vi "postData_bkp.vi"(7 "LabVIEW Web Service Request":refnum<class "Web Request.lvclass">) -> (2 "Result":string)   [LabVIEW 2016]
uses:
  <vilib>/wsapi/Web Request.lvclass
  <vilib>/Utility/file.llb/Read Delimited Spreadsheet (string).vi
  <vilib>/Utility/file.llb/Write Delimited Spreadsheet (string).vi
  <vilib>/Utility/file.llb/Read Delimited Spreadsheet (DBL).vi
  <vilib>/Utility/file.llb/Write Delimited Spreadsheet (DBL).vi
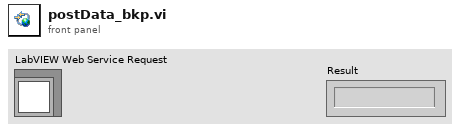
[diagram p1: front panel]
types:
  T1 = enum16{"open", "replace", "create", "open or create", "replace or create", "replace or create with confirmation"}
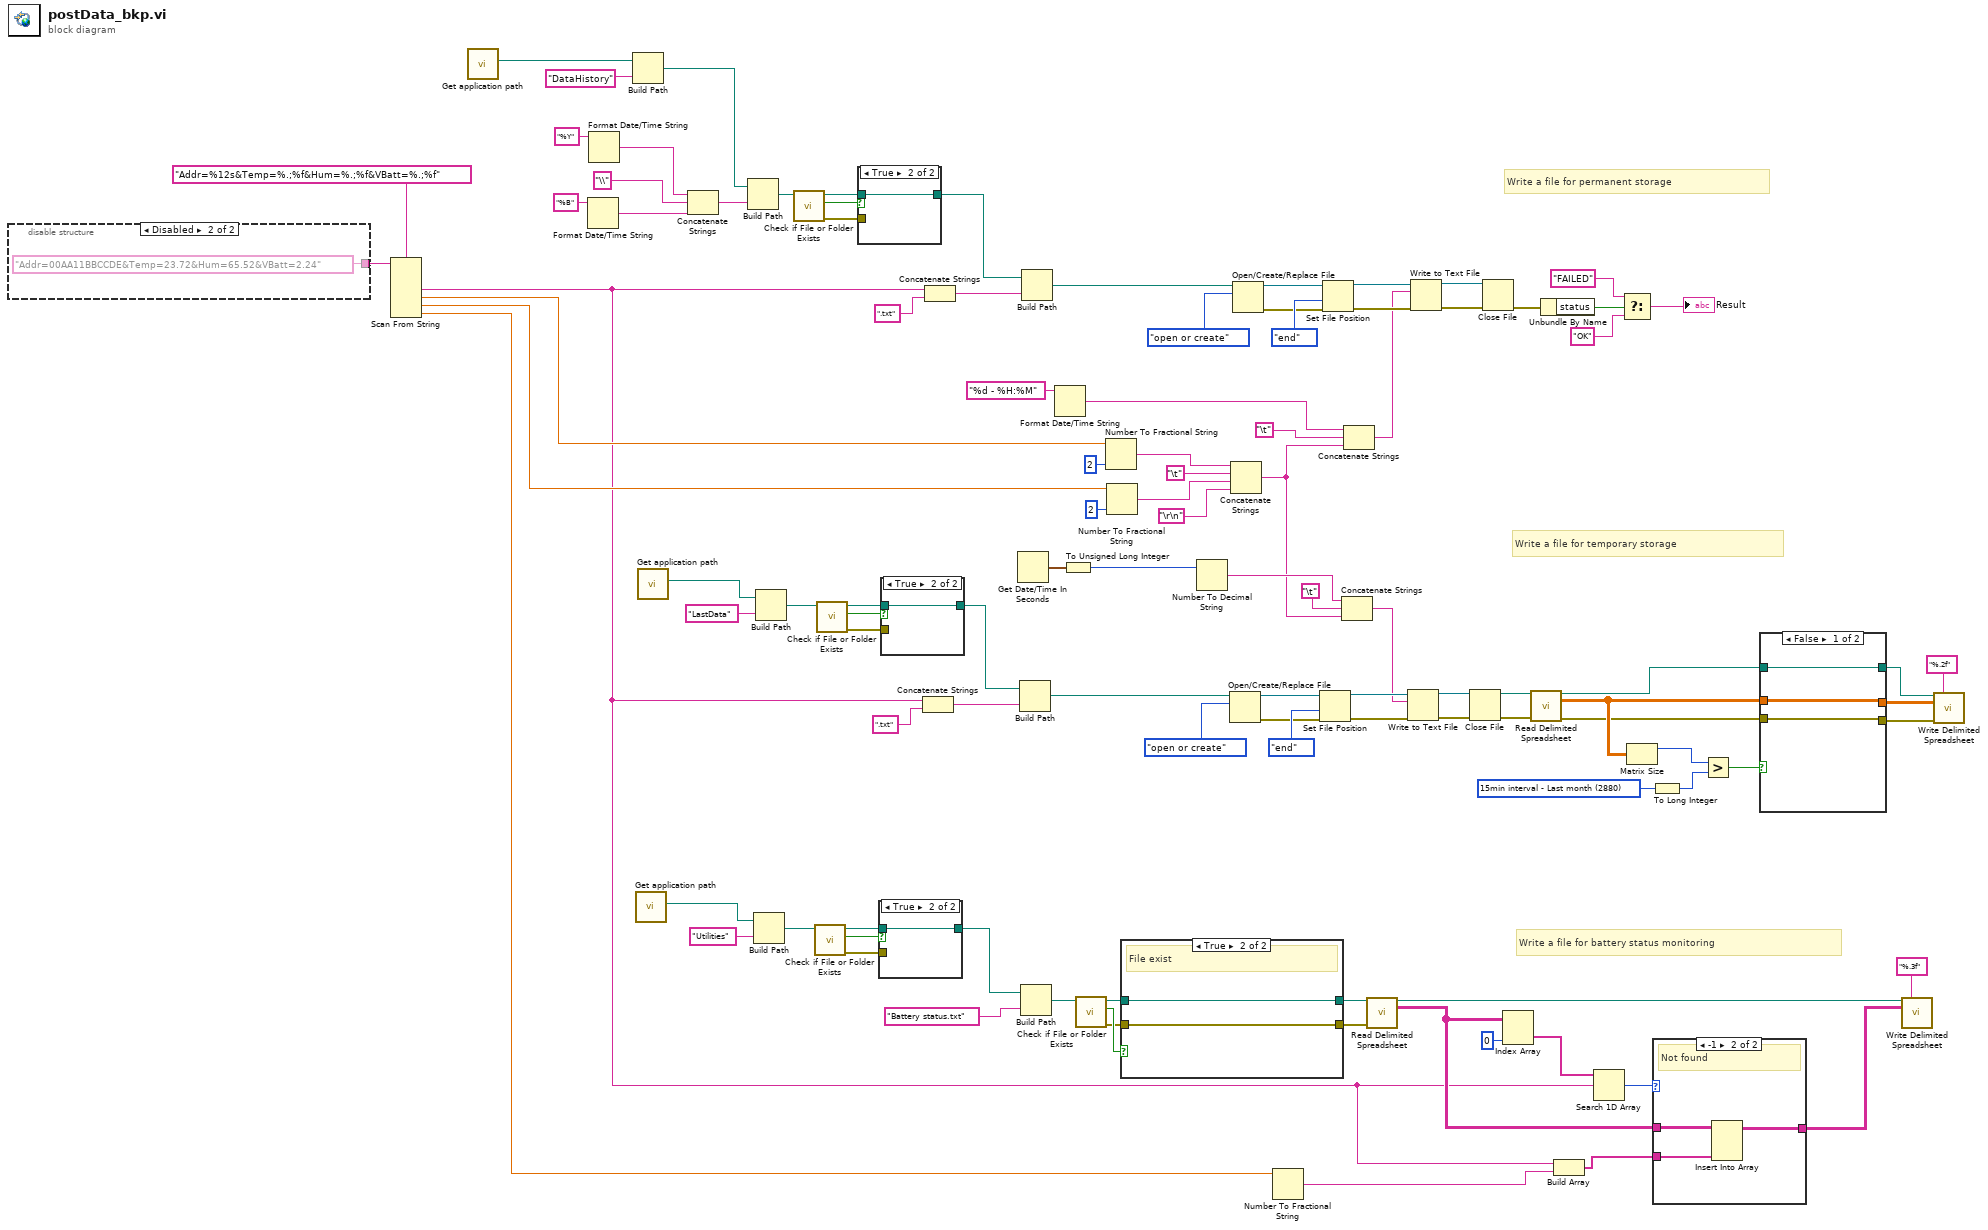
[diagram p0: block diagram]
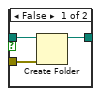
[diagram p2: hidden frame]
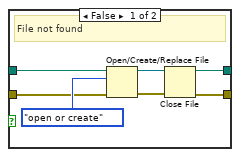
[diagram p3: hidden frame]
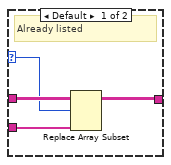
[diagram p4: hidden frame]
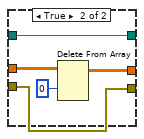
[diagram p5: hidden frame]
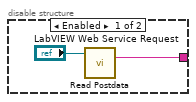
[diagram p6: hidden frame]
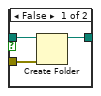
[diagram p7: hidden frame]
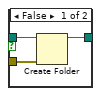
[diagram p8: hidden frame]
diagram:
  w11 = u16 2880 items=["5min interval - Last week"=2016, "5min interval - Last month"=8640, "10min interval - Last week"=1008, "10min interval - Last month"=4320, "15min interval - Last week"=672, "15min interval - Last month"=2880]
  # "Write a file for battery status monitoring"
  # "Write a file for temporary storage"
  # "Write a file for permanent storage"
  n1 = disable-structure shown="Disabled" {
    disable-tunnel: [w107 "Addr=00AA11BBCCDE&Temp=23.72&Hum=65.52&VBatt=2.24" ("input string")] -> w35
    frame Enabled {
      n2 = call <vilib>:"Read Postdata.vi"("LabVIEW Web Service Request"="LabVIEW Web Service Request") -> ("postdata"=w107:string)  [unwired: 12 in, 2 out]
    }
    frame Disabled {
    }
  }
  n3 = Scan From String(format string="Addr=%12s&Temp=%.;%f&Hum=%.;%f&VBatt=%.;%f", input string=w35) -> (output 1=w23:string, output 2=w88:dbl, output 3=w87:dbl, output 4=w22:dbl)  [unwired: 6 in, 3 out]
  n4 = call "Get application path.vi"() -> ("Application path"=w31:path)  [unwired: 11 in]
  n5 = Format Date/Time String(time format string (%c)="%B") -> (date/time string=w82:string)  [unwired: 2 in]
  n6 = Format Date/Time String(time format string (%c)="%Y") -> (date/time string=w84:string)  [unwired: 2 in]
  n7 = Build Path(base path=w31, name or relative path="DataHistory") -> (appended path=w34:path)
  n8 = call "Get application path.vi"() -> ("Application path"=w2:path)  [unwired: 11 in]
  n9 = call "Get application path.vi"() -> ("Application path"=w30:path)  [unwired: 11 in]
  n10 = Concatenate Strings(w84, "\\" ("string"), w82) -> (w89:string)
  n11 = Build Path(base path=w34, name or relative path=w89) -> (appended path=w80:path)
  n12 = Build Path(base path=w2, name or relative path="Utilities") -> (appended path=w7:path)
  n13 = Build Path(base path=w30, name or relative path="LastData") -> (appended path=w72:path)
  n14 = call <vilib>:"Check if File or Folder Exists.vi"("path"=w80) -> ("error out"=w79:errorcluster, "file or folder exists?"=w77:bool, "dup path"=w78:path)  [unwired: 8 in]
  n15 = call <vilib>:"Check if File or Folder Exists.vi"("path"=w7) -> ("error out"=w6:errorcluster, "file or folder exists?"=w4:bool, "dup path"=w5:path)  [unwired: 8 in]
  n16 = call <vilib>:"Check if File or Folder Exists.vi"("path"=w72) -> ("error out"=w71:errorcluster, "file or folder exists?"=w69:bool, "dup path"=w70:path)  [unwired: 8 in]
  n17 = case shown="True" w77 {
    tunnel: w79 -> [w112 _]
    tunnel: w78 -> [w111 w113]
    tunnel: [w110 w113] -> w76
    frame False {
      n18 = Create Folder(path (use dialog)=w111, error in=w112) -> (created path=w110:path)  [unwired: 1 in, 2 out]
    }
    frame True {
    }
  }
  n19 = case shown="True" w4 {
    tunnel: w6 -> [w116 _]
    tunnel: w5 -> [w115 w117]
    tunnel: [w114 w117] -> w1
    frame False {
      n20 = Create Folder(path (use dialog)=w115, error in=w116) -> (created path=w114:path)  [unwired: 1 in, 2 out]
    }
    frame True {
    }
  }
  n21 = case shown="True" w69 {
    tunnel: w71 -> [w120 _]
    tunnel: w70 -> [w119 w121]
    tunnel: [w118 w121] -> w29
    frame False {
      n22 = Create Folder(path (use dialog)=w119, error in=w120) -> (created path=w118:path)  [unwired: 1 in, 2 out]
    }
    frame True {
    }
  }
  n23 = Concatenate Strings(w23, ".txt" ("string")) -> (w67:string)
  n24 = Concatenate Strings(w23, ".txt" ("string")) -> (w74:string)
  n25 = Get Date/Time In Seconds() -> (seconds since 1Jan1904=w59:timestamp)
  n26 = Build Path(base path=w29, name or relative path=w67) -> (appended path=w60:path)
  n27 = Build Path(base path=w1, name or relative path="Battery status.txt" ("string")) -> (appended path=w15:path)
  n28 = Build Path(base path=w76, name or relative path=w74) -> (appended path=w73:path)
  n29 = Format Date/Time String(time format string (%c)="%d - %H:%M") -> (date/time string=w57:string)  [unwired: 2 in]
  n30 = To Unsigned Long Integer(number=w59) -> (unsigned 32bit integer=w51:u32)
  n31 = call <vilib>:"Check if File or Folder Exists.vi"("path"=w15) -> ("error out"=w12:errorcluster, "file or folder exists?"=w14:bool, "dup path"=w13:path)  [unwired: 8 in]
  n32 = Number To Fractional String(number=w88, precision (6)=i16 2) -> (F-format string=w106:string)  [unwired: 2 in]
  n33 = Number To Fractional String(number=w87, precision (6)=i16 2) -> (F-format string=w105:string)  [unwired: 2 in]
  n34 = case shown="True" w14 {
    tunnel: [w125 w130] -> w17
    tunnel: [w124 w129] -> w16
    tunnel: w13 -> [w123 w130]
    tunnel: w12 -> [w122 w129]
    frame False {
      # "File not found"
      n35 = Open/Create/Replace File(file path (use dialog)=w123, error in=w122, operation (0:open)=T1."open or create") -> (refnum out=w126:refnum<file>, error out=w127:errorcluster)  [unwired: 3 in, 1 out]
      n36 = Close File(refnum=w126, error in=w127) -> (path=w125:path, error out=w124:errorcluster)
    }
    frame True {
      # "File exist"
    }
  }
  n37 = Number To Decimal String(number=w51) -> (decimal integer string=w54:string)  [unwired: 1 in]
  n38 = Open/Create/Replace File(file path (use dialog)=w60, operation (0:open)=T1."open or create") -> (refnum out=w65:refnum<file>, error out=w63:errorcluster)  [unwired: 4 in, 1 out]
  n39 = Concatenate Strings(w106, "\t", w105, "\r\n") -> (w53:string)
  n40 = Open/Create/Replace File(file path (use dialog)=w73, operation (0:open)=T1."open or create") -> (refnum out=w94:refnum<file>, error out=w92:errorcluster)  [unwired: 4 in, 1 out]
  n41 = Number To Fractional String(number=w22) -> (F-format string=w21:string)  [unwired: 3 in]
  n42 = Set File Position(refnum=w65, from (0:start)=enum16{"start", "end", "current"}."end", error in=w63) -> (refnum out=w61:refnum<file>, error out=w62:errorcluster)  [unwired: 1 in]
  n43 = Set File Position(refnum=w94, from (0:start)=enum16{"start", "end", "current"}."end", error in=w92) -> (refnum out=w90:refnum<file>, error out=w91:errorcluster)  [unwired: 1 in]
  n44 = Concatenate Strings(w54, "\t", w53) -> (w52:string)
  n45 = Concatenate Strings(w57, "\t", w53) -> (w56:string)
  n46 = call-poly <vilib>:"Read Delimited Spreadsheet.vi"("file path (dialog if empty)"=w17, "error in (no error)"=w16) -> ("new file path (Not A Path if cancelled)"=w19:path, "all rows"=w24:string[][])  [unwired: 8 in, 4 out]
  n47 = Write to Text File(file (use dialog)=w61, text=w52, error in=w62) -> (refnum out=w50:refnum<file>, error out=w49:errorcluster)  [unwired: 1 in, 1 out]
  n48 = Write to Text File(file (use dialog)=w90, text=w56, error in=w91) -> (refnum out=w102:refnum<file>, error out=w101:errorcluster)  [unwired: 1 in, 1 out]
  n49 = Close File(refnum=w50, error in=w49) -> (path=w40:path, error out=w39:errorcluster)
  n50 = Close File(refnum=w102, error in=w101) -> (error out=w99:errorcluster)  [unwired: 1 out]
  n51 = Index Array(array=w24, index (col)=0 ("disabled index (col)")) -> (element=w26:string[])  [unwired: 1 in]
  n52 = call-poly <vilib>:"Read Delimited Spreadsheet.vi"("file path (dialog if empty)"=w40, "error in (no error)"=w39) -> ("new file path (Not A Path if cancelled)"=w43:path, "all rows"=w45:dbl[][], "error out"=w41:errorcluster)  [unwired: 8 in, 3 out]
  n53 = Unbundle By Name(w99) -> ("status"=w98:bool)
  n54 = Build Array(w23, w21) -> (w20:string[])
  n55 = Search 1D Array(1D array=w26, element=w23) -> (index of element=w25:i32)  [unwired: 1 in]
  n56 = Select(t="FAILED", s=w98, f="OK") -> (s? t:f=→"Result":string)
  n57 = Matrix Size(0:w45) -> (1:w48:i32)  [unwired: 1 out]
  n58 = To Long Integer(number=w11) -> (32bit integer=w10:i32)
  n59 = case shown="-1" w25 {
    selector: w25 -> [w132 _]
    tunnel: w24 -> [w134 w137]
    tunnel: w20 -> [w133 w136]
    tunnel: [w131 w135] -> w18
    frame Default {
      # "Already listed"
      n60 = Replace Array Subset(array=w134, new element=w133, index (row)=w132) -> (w131:string[][])  [unwired: 1 in]
    }
    frame -1 {
      # "Not found"
      n61 = Insert Into Array(array=w137, new element=w136) -> (w135:string[][])  [unwired: 2 in]
    }
  }
  n62 = Greater?(x=w48, y=w10) -> (0:w47:bool)
  n63 = case shown="False" w47 {
    tunnel: w45 -> [w140 w145]
    tunnel: [w140 w143] -> w46
    tunnel: [w139 w142] -> w44
    tunnel: w43 -> [w139 w142]
    tunnel: [w138 w141] -> w42
    tunnel: w41 -> [w138 w141]
    frame False {
    }
    frame True {
      n64 = Delete From Array(array=w145, index (row)=0) -> (array with subset deleted=w143:dbl[][])  [unwired: 2 in, 1 out]
    }
  }
  n65 = call-poly <vilib>:"Write Delimited Spreadsheet.vi"("file path (dialog if empty)"=w19, "format (%s)"="%.3f" ("format (%.3f)"), "2D data"=w18) -> ()  [unwired: 11 in, 2 out]
  n66 = call-poly <vilib>:"Write Delimited Spreadsheet.vi"("file path (dialog if empty)"=w44, "format (%.3f)"="%.2f", "2D data"=w46, "error in (no error)"=w42) -> ()  [unwired: 10 in, 2 out]
